vi "Event Generate Event.vi"(4 "Video Modes":string[](array[string]), 6 "Camera Name":string, 9 "Setpoint":i64, 11 "Event Type":T1=enum."Save Data") -> ()   [LabVIEW 2023]
uses:
  Event Setup Types.ctl
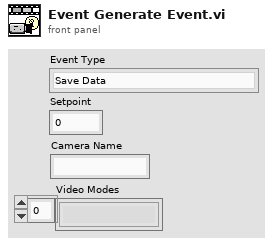
[diagram p1: front panel]
types:
  T1 = typedef "Event Setup Types.ctl" = enum16{"Default", "Camera Loop Started", "Close Settings", "GreyScale", "Open Front Panel", "Reset Team Number", "Save Data", "Exit"}
  T2 = typedef "Camera Event Cluster.ctl" = cluster{"Event Type":T1, "Setpoint":i64, "Camera":string, "Video Modes":string[]}
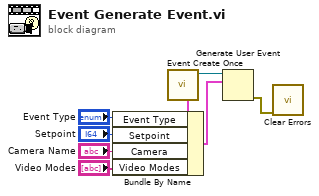
[diagram p0: block diagram]
diagram:
  n1 = call "Event Create Once.vi"() -> ("Camera Events"=w8:refnum<user-event>, "Camera Events 2"=w7:T2)  [unwired: 10 in]
  n2 = Bundle By Name(cluster=w7, "Event Type"="Event Type", "Setpoint"="Setpoint", "Camera"="Camera Name", "Video Modes"="Video Modes") -> (w6:T2)
  n3 = Generate User Event(user event=w8, event data cluster=w6) -> (error out=w1:errorcluster)  [unwired: 2 in, 1 out]
  n4 = call <vilib>:"Clear Errors.vi"("error in (no error)"=w1) -> ()  [unwired: 5 in, 2 out]
